vi "Main_v1.2.1.vi"() -> ()   [LabVIEW 2018]
uses:
  <vilib>/Utility/error.llb/DialogType.ctl
panel:
  out "字符串":string
  out "Progress Bar":i32(slide) max=135 scale=1.0..2026.0
  out "结果":T1(plugin-control)
  out "识别螺旋桨":T1(plugin-control)
  out "识别空泡":T1(plugin-control)
  in  "停止按钮":bool
  in  "等待时间（毫秒）":u32=100
  in  "打开按钮":bool
  # "空泡智能识别系统"
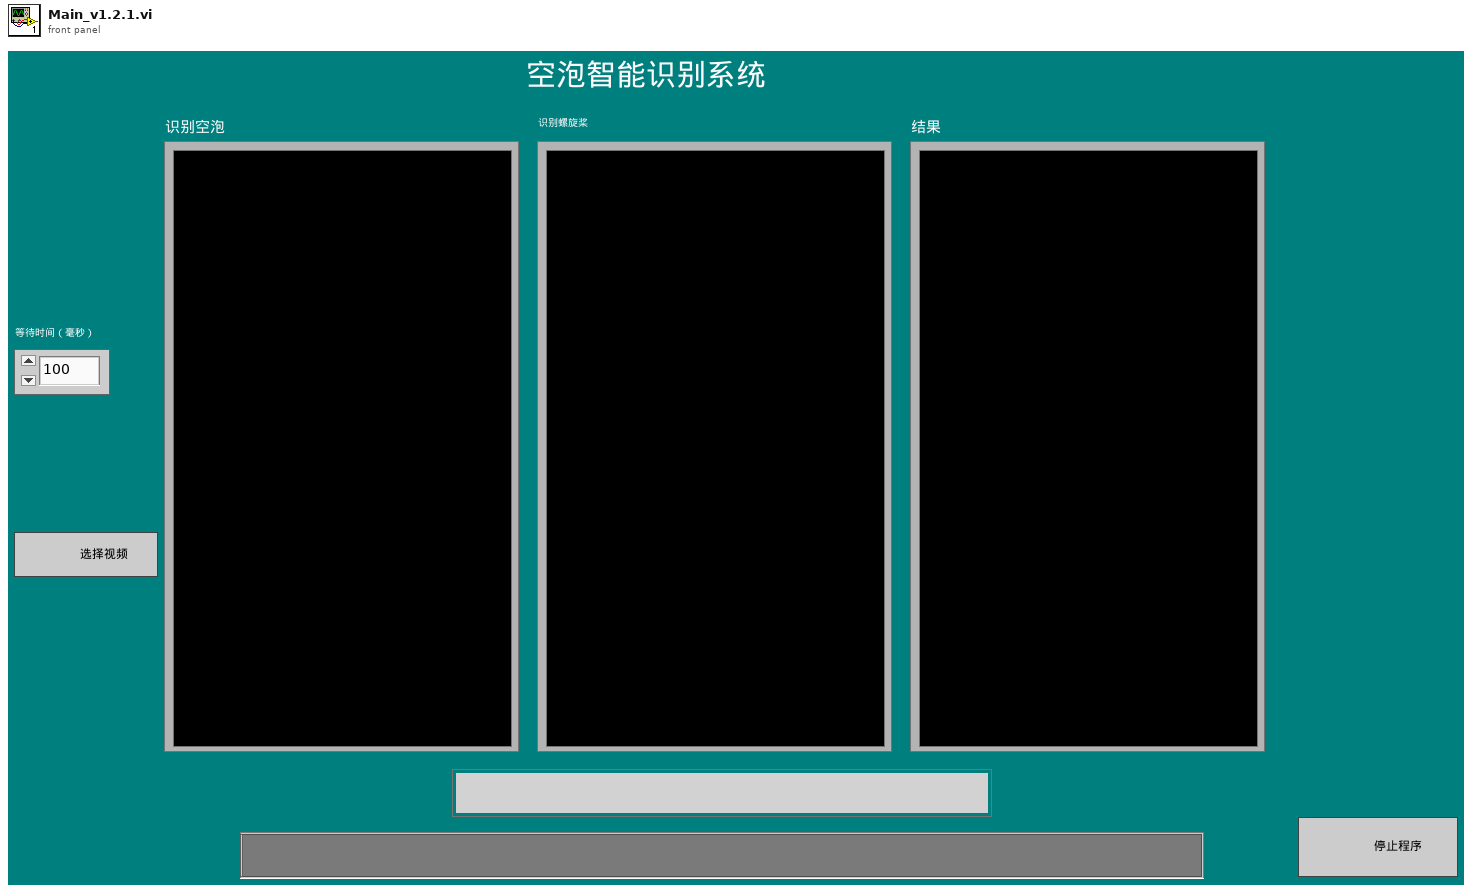
[diagram p1: front panel]
types:
  T1 = typedef "IMAQ Image.ctl" = refnum<image>
  T2 = cluster{"Desired Font (Application)":enum16{"User-specified Font", "Application Font", "System Font", "Dialog Font"}, "[User-specified Font]":cluster{"Font Name":string, "Size":i16, "Strikeout?":bool, "Italic?":bool, "Underline?":bool, "Outline?":bool, "Shadow?":bool, "Bold?":bool, "Rotation Angle":dbl}, "Horizontal Alignment":i16, "Vertical Alignment":i16}
  T3 = typedef "IMAQ AVI2 Refnum.ctl" = refnum<k20>
  T4 = typedef "Image Type" = u32
  T5 = cluster{"Width":u32, "Height":u32, "Frames Per Second":u32, "Codec":string, "Has Data":bool}
  T6 = typedef "DialogType.ctl" = u16
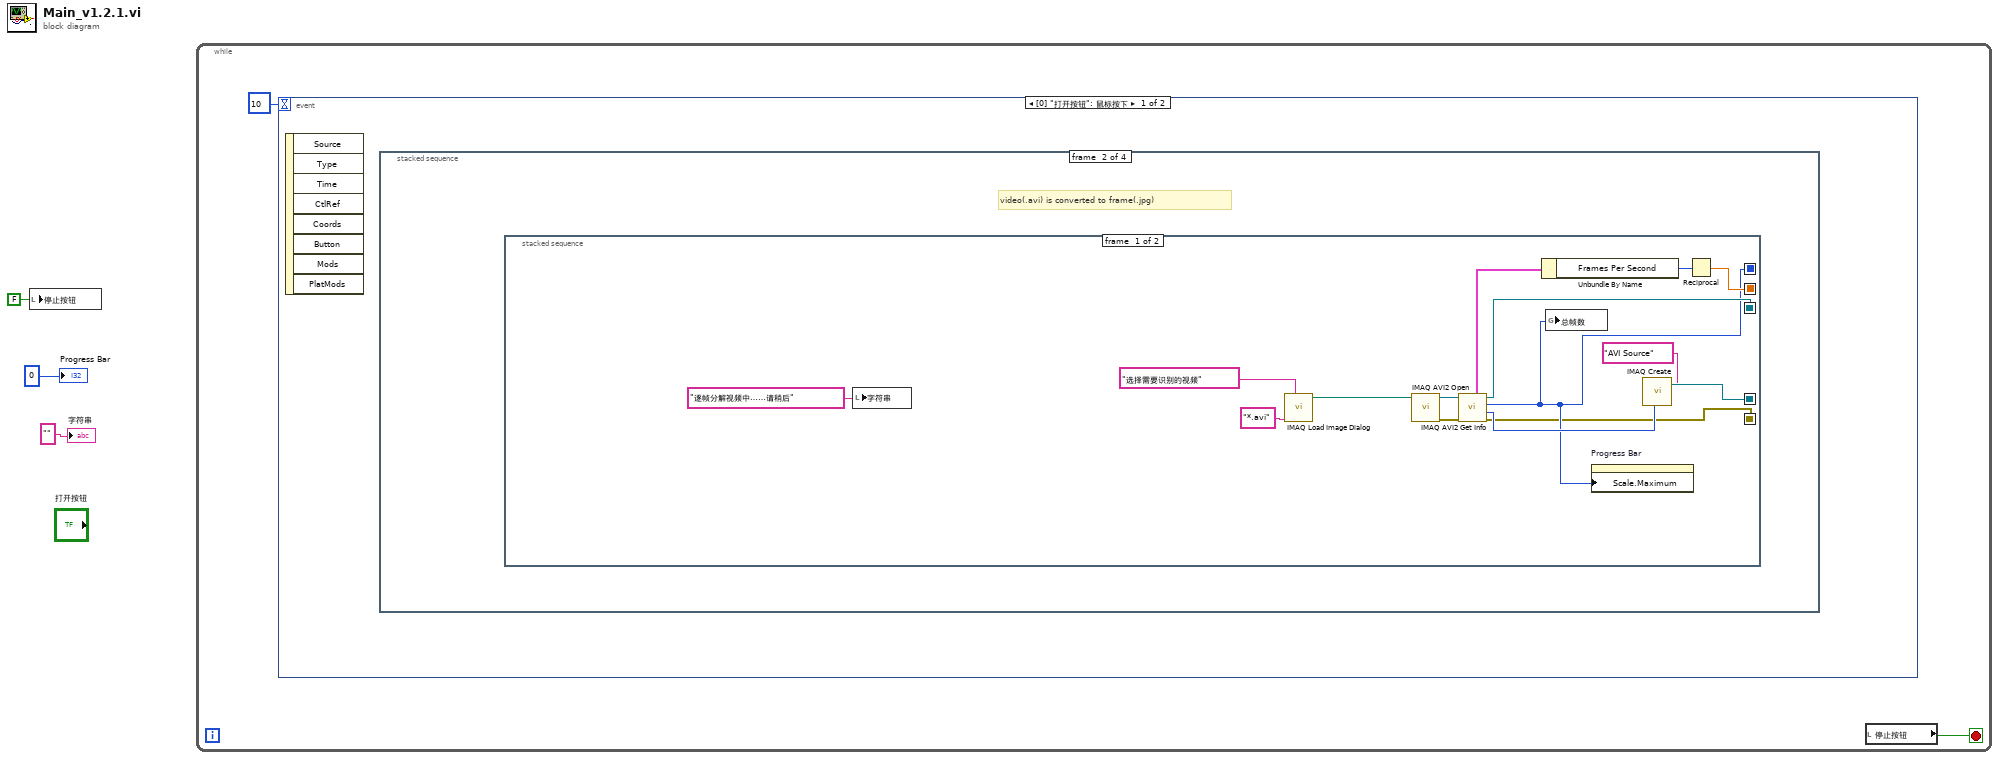
[diagram p0: block diagram]
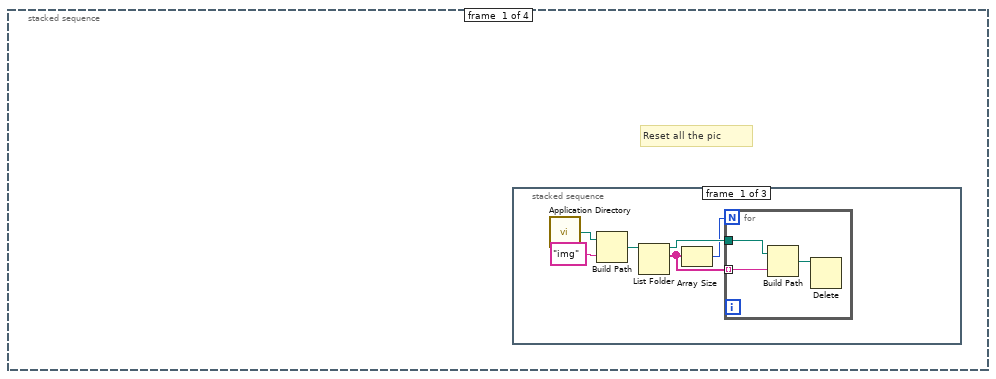
[diagram p2: hidden frame]
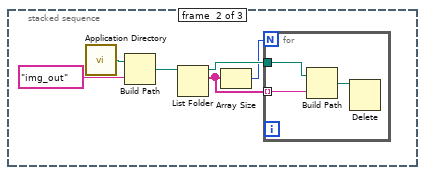
[diagram p3: hidden frame]
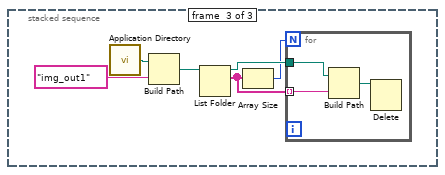
[diagram p4: hidden frame]
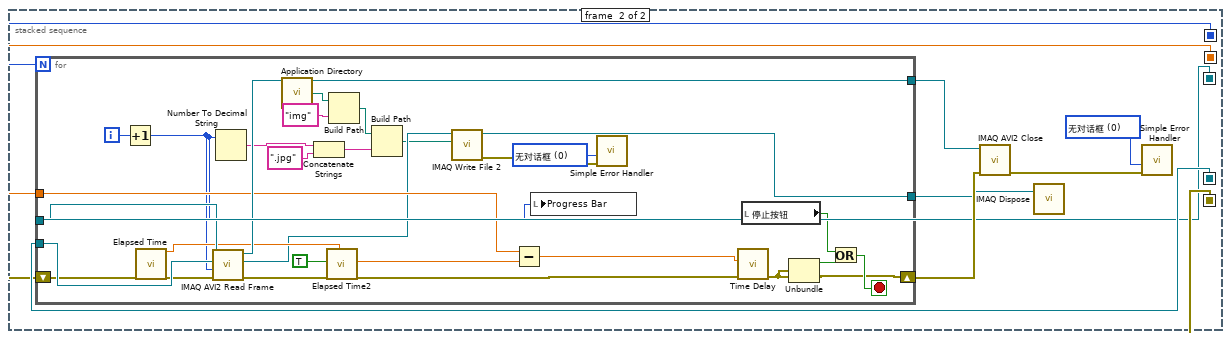
[diagram p5: hidden frame]
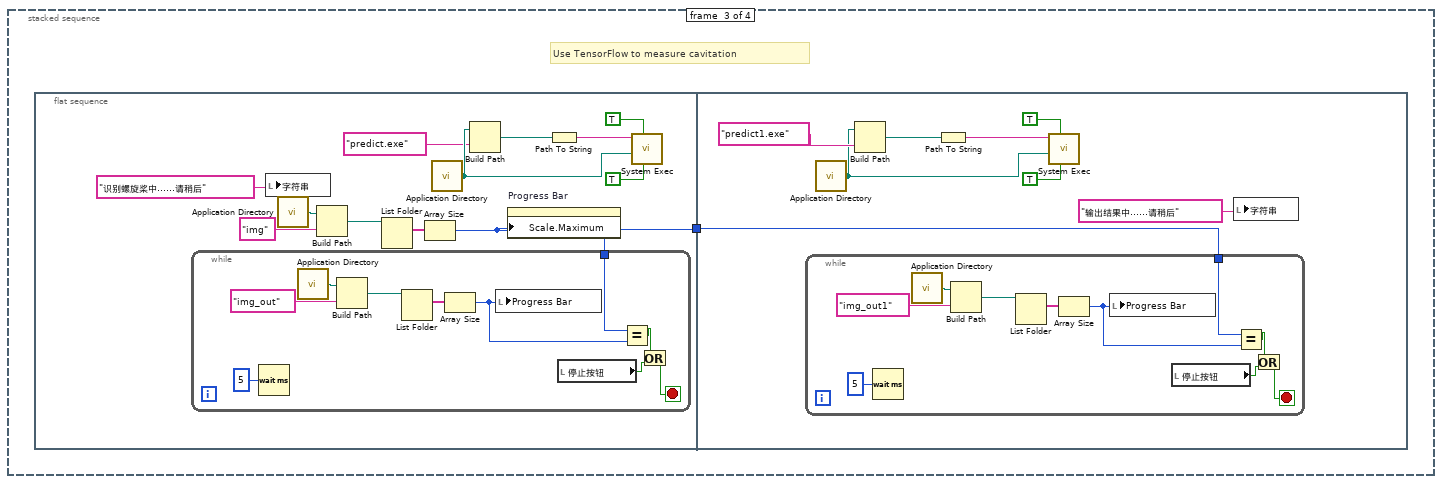
[diagram p6: hidden frame]
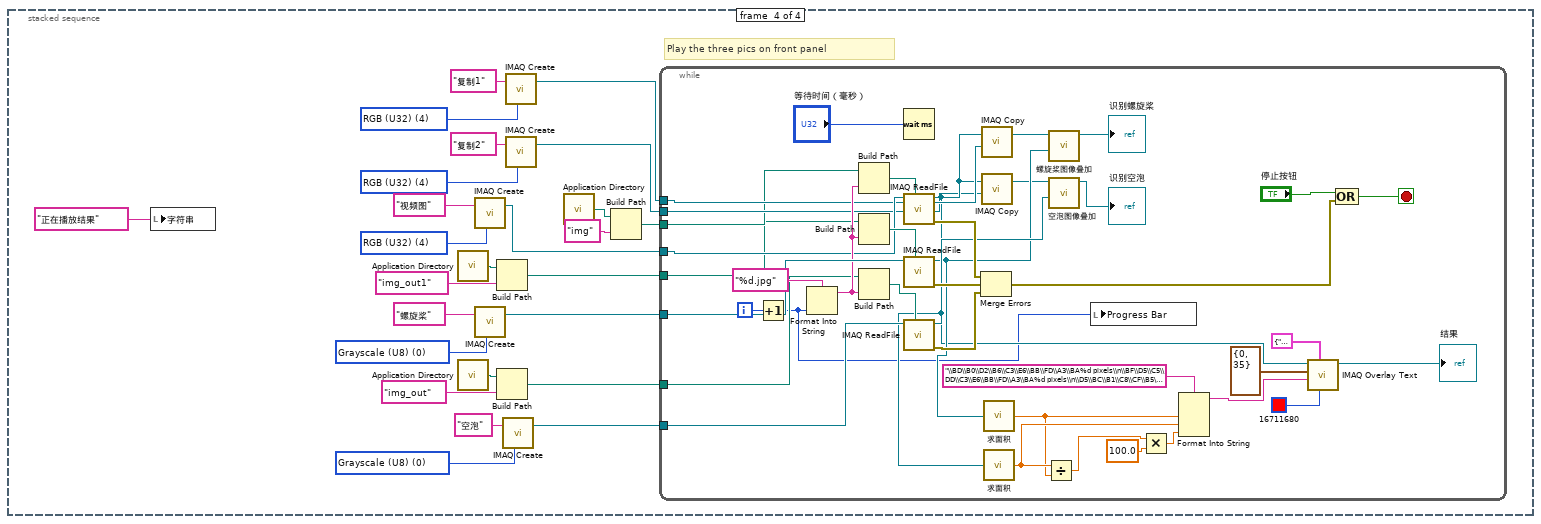
[diagram p7: hidden frame]
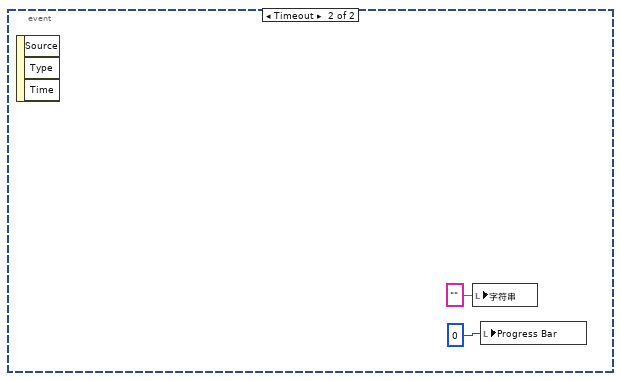
[diagram p8: hidden frame]
diagram:
  n1 = local write "停止按钮"(FALSE ("停止按钮")) -> ()
  n2 = while {
    stop <- w5 stop-if-true
    n3 = event shown="[0] \"打开按钮\": 鼠标按下" {
      selector: _ -> [_ _]
      dyn-events: _ -> [_ _]
      timeout: 10 -> [_ _]
      event "打开按钮": Mouse Down {
        n4 = event-data() -> ()  [unwired: 1 in, 8 out]
        n5 = stacked-sequence {
          frame #0 {
            # "Reset all the pic"
            n6 = stacked-sequence {
              frame #0 {
                n7 = call <vilib>:"Application Directory.vi"() -> ("Application Directory"=w10:path)
                n8 = Build Path(base path=w10, name or relative path="img" ("名称或相对路径")) -> (appended path=w8:path)
                n9 = List Folder(path=w8) -> (path out=w11:path, filenames=w6:string[])  [unwired: 3 in, 2 out]
                n10 = Array Size(array=w6) -> (size(s)=w7:i32)
                n11 = for {
                  N: w7 -> [_]
                  tunnel: w11 -> [w13]
                  tunnel: w6 -> [w12] mode=indexing
                  n12 = Build Path(base path=w13, name or relative path=w12) -> (appended path=w14:path)
                  n13 = Delete(path (use dialog)=w14) -> ()  [unwired: 4 in, 3 out]
                }
              }
              frame #1 {
                n14 = call <vilib>:"Application Directory.vi"() -> ("Application Directory"=w19:path)
                n15 = Build Path(base path=w19, name or relative path="img_out" ("名称或相对路径")) -> (appended path=w17:path)
                n16 = List Folder(path=w17) -> (path out=w20:path, filenames=w15:string[])  [unwired: 3 in, 2 out]
                n17 = Array Size(array=w15) -> (size(s)=w16:i32)
                n18 = for {
                  N: w16 -> [_]
                  tunnel: w20 -> [w22]
                  tunnel: w15 -> [w21] mode=indexing
                  n19 = Build Path(base path=w22, name or relative path=w21) -> (appended path=w23:path)
                  n20 = Delete(path (use dialog)=w23) -> ()  [unwired: 4 in, 3 out]
                }
              }
              frame #2 {
                n21 = call <vilib>:"Application Directory.vi"() -> ("Application Directory"=w28:path)
                n22 = Build Path(base path=w28, name or relative path="img_out1" ("名称或相对路径")) -> (appended path=w26:path)
                n23 = List Folder(path=w26) -> (path out=w29:path, filenames=w25:string[])  [unwired: 3 in, 2 out]
                n24 = Array Size(array=w25) -> (size(s)=w24:i32)
                n25 = for {
                  N: w24 -> [_]
                  tunnel: w29 -> [w31]
                  tunnel: w25 -> [w30] mode=indexing
                  n26 = Build Path(base path=w31, name or relative path=w30) -> (appended path=w32:path)
                  n27 = Delete(path (use dialog)=w32) -> ()  [unwired: 4 in, 3 out]
                }
              }
            }
          }
          frame #1 {
            # "video(.avi) is converted to frame(.jpg)"
            n28 = stacked-sequence {
              seq-local: [w35 _] -> [_ w49]
              seq-local: [w34 _] -> [_ w52]
              seq-local: [w44 _] -> [_ w53]
              seq-local: [w43 _] -> [_ w51]
              seq-local: [w40 _] -> [_ w50]
              frame #0 {
                n29 = local write "字符串"("逐帧分解视频中……请稍后" ("字符串")) -> ()
                n30 = call "IMAQ Load Image Dialog"("Prompt"="选择需要识别的视频" ("prompt"), "Pattern"="*.avi") -> ("Path"=w39:path)  [unwired: 7 in, 2 out]
                n31 = call "IMAQ AVI2 Open"("AVI File Path"=w39) -> ("error out"=w46:errorcluster, "AVI Refnum"=w45:T3)  [unwired: 2 in, 7 out]
                n32 = call "IMAQ AVI2 Get Info"("error in (no error)"=w46, "AVI Refnum"=w45) -> ("error out"=w34:errorcluster, "Image Type"=w42:T4, "Number of Frames"=w35:u32, "AVI Refnum (duplicate)"=w43:T3, "Frame Data"=w47:T5)  [unwired: 5 out]
                n33 = Unbundle By Name(w47) -> ("Frames Per Second"=w41:u32)
                n34 = global write "全局变量.vi" "总帧数"(w35) -> ()
                n35 = property on="Progress Bar" class="Slide (严格)"("Scale.Maximum"=w35) -> ()  [unwired: 2 in, 2 out]
                n36 = call "IMAQ Create"("Image Name"="AVI Source", "Image Type"=w42) -> ("New Image"=w44:T1)  [unwired: 2 in, 2 out]
                n37 = Reciprocal(x=w41) -> (1/x=w40:dbl)
              }
              frame #1 {
                w54 = T6 0 items=["无对话框", "确定信息", "继续或停止信息", "确定信息＋警告", "继续/停止+警告"] ("type of dialog (OK msg:1)")
                n38 = for "For循环" {
                  N: w49 -> [_]
                  tunnel: [w84] -> w57
                  tunnel: w51 -> [w86]
                  tunnel: w50 -> [w81]
                  shift-right: [w62] -> w56
                  shift-left: w52 -> [w83]
                  tunnel: w53 -> [w85]
                  tunnel: [w60] -> w48
                  i -> [w66]
                  stop <- w64 stop-if-true
                  w58 = T6 0 items=["无对话框", "确定信息", "继续或停止信息", "确定信息＋警告", "继续/停止+警告"] ("type of dialog (OK msg:1)")
                  n39 = Increment(x=w66) -> (x+1=w65:i32)
                  n40 = call "Elapsed Time"("error in (no error)"=w83) -> ("Present (s)"=w79:dbl, "error out"=w82:errorcluster)  [unwired: 11 in, 6 out]
                  n41 = call "IMAQ AVI2 Read Frame"("error in (no error)"=w82, "Frame Number"=w65, "Image"=w85, "AVI Refnum"=w86) -> ("error out"=w77:errorcluster, "Image Out"=w74:T1, "AVI Refnum (duplicate)"=w84:T3)  [unwired: 5 out]
                  n42 = Number To Decimal String(number=w65) -> (decimal integer string=w69:string)  [unwired: 1 in]
                  n43 = call <vilib>:"Application Directory.vi"() -> ("Application Directory"=w73:path)
                  n44 = Concatenate Strings(w69, ".jpg" ("字符串")) -> (w67:string)
                  n45 = call "Elapsed Time2"("Reset"=TRUE, "error in (no error)"=w77, "Set Start Time (s)"=w79) -> ("Elapsed Time (s)"=w76:dbl, "error out"=w75:errorcluster)  [unwired: 9 in, 6 out]
                  n46 = Build Path(base path=w73, name or relative path="img" ("名称或相对路径")) -> (appended path=w71:path)
                  n47 = Build Path(base path=w71, name or relative path=w67) -> (appended path=w70:path)
                  n48 = call-poly "IMAQ Write File 2"("File Path"=w70, "Image"=w74) -> ("error out"=w59:errorcluster, "Image Out (duplicate)"=w60:T1)  [unwired: 8 in]
                  n49 = Subtract(x=w81, y=w76) -> (x-y=w80:dbl)
                  n50 = local write "Progress Bar"(w65) -> ()
                  n51 = call <vilib>:"Simple Error Handler.vi"("type of dialog (OK msg:1)"=w58, "error in (no error)"=w59) -> ()  [unwired: 3 in, 5 out]
                  n52 = call "Time Delay"("error in (no error)"=w75, "Delay Time (s)"=w80) -> ("error out"=w62:errorcluster)  [unwired: 9 in]
                  n53 = local read "停止按钮"() -> (w63:bool)
                  n54 = Unbundle(w62) -> ("status"=w61:bool)  [unwired: 2 out]
                  n55 = Or(x=w63, y=w61) -> (x .or. y?=w64:bool)
                }
                n56 = call "IMAQ AVI2 Close"("error in (no error)"=w56, "AVI Refnum"=w57) -> ("error out"=w55:errorcluster)  [unwired: 9 out]
                n57 = call "IMAQ Dispose"("Image"=w48) -> ()  [unwired: 2 in, 4 out]
                n58 = call <vilib>:"Simple Error Handler.vi"("type of dialog (OK msg:1)"=w54, "error in (no error)"=w55) -> ()  [unwired: 8 out]
              }
            }
          }
          frame #2 {
            # "Use TensorFlow to measure cavitation"
            n59 = flat-sequence {
              tunnel: [w88] -> w87
              tunnel: w87 -> [w110]
              frame #0 {
                n60 = local write "字符串"("识别螺旋桨中……请稍后" ("字符串")) -> ()
                n61 = call <vilib>:"Application Directory.vi"() -> ("Application Directory"=w90:path)
                n62 = Build Path(base path=w90, name or relative path="img" ("名称或相对路径")) -> (appended path=w91:path)
                n63 = List Folder(path=w91) -> (filenames=w89:string[])  [unwired: 3 in, 3 out]
                n64 = Array Size(array=w89) -> (size(s)=w88:i32)
                n65 = while {
                  tunnel: w88 -> [w103]
                  stop <- w100 stop-if-true
                  n66 = Wait (ms)(milliseconds to wait=u32 5 ("等待时间（毫秒）")) -> ()  [unwired: 1 out]
                  n67 = call <vilib>:"Application Directory.vi"() -> ("Application Directory"=w108:path)
                  n68 = Build Path(base path=w108, name or relative path="img_out" ("名称或相对路径")) -> (appended path=w107:path)
                  n69 = List Folder(path=w107) -> (filenames=w109:string[])  [unwired: 3 in, 3 out]
                  n70 = Array Size(array=w109) -> (size(s)=w104:i32)
                  n71 = local write "Progress Bar"(w104) -> ()
                  n72 = local read "停止按钮"() -> (w102:bool)
                  n73 = Equal?(x=w103, y=w104) -> (x = y?=w101:bool)
                  n74 = Or(x=w101, y=w102) -> (x .or. y?=w100:bool)
                }
                n75 = call <vilib>:"Application Directory.vi"() -> ("Application Directory"=w97:path)
                n76 = Build Path(base path=w97, name or relative path="predict.exe" ("名称或相对路径")) -> (appended path=w95:path)
                n77 = property on="Progress Bar" class="Slide (严格)"("Scale.Maximum"=w88) -> ()  [unwired: 2 in, 2 out]
                n78 = Path To String(path=w95) -> (string=w94:string)
                n79 = call <vilib>:"System Exec.vi"("run minimized? (F)"=TRUE, "wait until completion? (T)"=TRUE, "working directory"=w97, "command line"=w94) -> ()  [unwired: 4 in, 4 out]
              }
              frame #1 {
                n80 = while {
                  tunnel: w110 -> [w121]
                  stop <- w118 stop-if-true
                  n81 = Wait (ms)(milliseconds to wait=u32 5 ("等待时间（毫秒）")) -> ()  [unwired: 1 out]
                  n82 = call <vilib>:"Application Directory.vi"() -> ("Application Directory"=w126:path)
                  n83 = Build Path(base path=w126, name or relative path="img_out1" ("名称或相对路径")) -> (appended path=w125:path)
                  n84 = List Folder(path=w125) -> (filenames=w127:string[])  [unwired: 3 in, 3 out]
                  n85 = Array Size(array=w127) -> (size(s)=w122:i32)
                  n86 = local write "Progress Bar"(w122) -> ()
                  n87 = local read "停止按钮"() -> (w120:bool)
                  n88 = Equal?(x=w121, y=w122) -> (x = y?=w119:bool)
                  n89 = Or(x=w119, y=w120) -> (x .or. y?=w118:bool)
                }
                n90 = call <vilib>:"Application Directory.vi"() -> ("Application Directory"=w112:path)
                n91 = Build Path(base path=w112, name or relative path="predict1.exe" ("名称或相对路径")) -> (appended path=w114:path)
                n92 = Path To String(path=w114) -> (string=w113:string)
                n93 = call <vilib>:"System Exec.vi"("run minimized? (F)"=TRUE, "wait until completion? (T)"=TRUE, "working directory"=w112, "command line"=w113) -> ()  [unwired: 4 in, 4 out]
                n94 = local write "字符串"("输出结果中……请稍后" ("字符串")) -> ()
              }
            }
          }
          frame #3 {
            w140 = T4 4 items=["Grayscale (U8)", "Grayscale (I16)", "Grayscale (SGL)", "Complex (CSG)", "RGB (U32)", "HSL (U32)", "RGB (U64)", "Grayscale (U16)"] ("Image Type")
            w143 = T4 4 items=["Grayscale (U8)", "Grayscale (I16)", "Grayscale (SGL)", "Complex (CSG)", "RGB (U32)", "HSL (U32)", "RGB (U64)", "Grayscale (U16)"] ("Image Type")
            w146 = T4 0 items=["Grayscale (U8)", "Grayscale (I16)", "Grayscale (SGL)", "Complex (CSG)", "RGB (U32)", "HSL (U32)", "RGB (U64)", "Grayscale (U16)"] ("Image Type")
            w149 = T4 0 items=["Grayscale (U8)", "Grayscale (I16)", "Grayscale (SGL)", "Complex (CSG)", "RGB (U32)", "HSL (U32)", "RGB (U64)", "Grayscale (U16)"] ("Image Type")
            w151 = T4 4 items=["Grayscale (U8)", "Grayscale (I16)", "Grayscale (SGL)", "Complex (CSG)", "RGB (U32)", "HSL (U32)", "RGB (U64)", "Grayscale (U16)"] ("Image Type")
            # "Play the three pics on front panel"
            n95 = local write "字符串"("正在播放结果" ("字符串")) -> ()
            n96 = call <vilib>:"Application Directory.vi"() -> ("Application Directory"=w131:path)
            n97 = call <vilib>:"Application Directory.vi"() -> ("Application Directory"=w133:path)
            n98 = call "IMAQ Create"("Image Name"="视频图", "Image Type"=w151) -> ("New Image"=w150:T1)  [unwired: 3 in, 1 out]
            n99 = call "IMAQ Create"("Image Name"="螺旋桨", "Image Type"=w149) -> ("New Image"=w144:T1)  [unwired: 3 in, 1 out]
            n100 = Build Path(base path=w131, name or relative path="img_out1" ("名称或相对路径")) -> (appended path=w129:path)
            n101 = Build Path(base path=w133, name or relative path="img_out" ("名称或相对路径")) -> (appended path=w132:path)
            n102 = call "IMAQ Create"("Image Name"="空泡", "Image Type"=w146) -> ("New Image"=w145:T1)  [unwired: 3 in, 1 out]
            n103 = call "IMAQ Create"("Image Name"="复制1", "Image Type"=w143) -> ("New Image"=w139:T1)  [unwired: 3 in, 1 out]
            n104 = call "IMAQ Create"("Image Name"="复制2", "Image Type"=w140) -> ("New Image"=w138:T1)  [unwired: 3 in, 1 out]
            n105 = call <vilib>:"Application Directory.vi"() -> ("Application Directory"=w137:path)
            n106 = Build Path(base path=w137, name or relative path="img" ("名称或相对路径")) -> (appended path=w135:path)
            n107 = while {
              tunnel: w150 -> [w164]
              tunnel: w145 -> [w186]
              tunnel: w144 -> [w185]
              tunnel: w139 -> [w162]
              tunnel: w138 -> [w160]
              tunnel: w135 -> [w156]
              tunnel: w132 -> [w155]
              tunnel: w129 -> [w154]
              i -> [w175]
              stop <- w168 stop-if-true
              n108 = Increment(x=w175) -> (x+1=w153:i32)
              n109 = Format Into String(format string="%d.jpg" ("格式字符串"), w153) -> (resulting string=w174:string)  [unwired: 2 in, 1 out]
              n110 = Build Path(base path=w156, name or relative path=w174) -> (appended path=w187:path)
              n111 = Build Path(base path=w154, name or relative path=w174) -> (appended path=w184:path)
              n112 = Build Path(base path=w155, name or relative path=w174) -> (appended path=w183:path)
              n113 = Wait (ms)(milliseconds to wait="等待时间（毫秒）") -> ()  [unwired: 1 out]
              n114 = call "IMAQ ReadFile"("File Path"=w187, "Image"=w164) -> ("error out"=w171:errorcluster, "Image Out"=w161:T1)  [unwired: 5 in, 3 out]
              n115 = call "IMAQ ReadFile"("File Path"=w184, "Image"=w185) -> ("error out"=w170:errorcluster, "Image Out"=w163:T1)  [unwired: 5 in, 3 out]
              n116 = call "IMAQ ReadFile"("File Path"=w183, "Image"=w186) -> ("error out"=w169:errorcluster, "Image Out"=w166:T1)  [unwired: 5 in, 3 out]
              n117 = Merge Errors(w171, w170, w169) -> (w172:errorcluster)
              n118 = call "IMAQ Copy"("Image Dst"=w162, "Image Src"=w161) -> ("Image Dst Out"=w158:T1)  [unwired: 4 in, 1 out]
              n119 = call "IMAQ Copy"("Image Dst"=w160, "Image Src"=w161) -> ("Image Dst Out"=w159:T1)  [unwired: 4 in, 1 out]
              n120 = call "求面积.vi"("Image"=w163) -> ("数值输入控件"=w181:dbl)
              n121 = call "求面积.vi"("Image"=w166) -> ("数值输入控件"=w182:dbl)
              n122 = Divide(x=w182, y=w181) -> (x/y=w180:dbl)
              n123 = call "螺旋桨图像叠加.vi"("Image Src A"=w163, "Image Src"=w158) -> ("Image Dst Out"=→"识别螺旋桨":T1)  [unwired: 9 in]
              n124 = call "空泡图像叠加.vi"("Image Src A"=w166, "Image Src"=w159) -> ("Image Dst Out"=→"识别空泡":T1)  [unwired: 9 in]
              n125 = local write "Progress Bar"(w153) -> ()
              n126 = Multiply(x=w180, y=100.0) -> (x*y=w178:dbl)
              n127 = Format Into String(format string="\\BD\\B0\\D2\\B6\\C3\\E6\\BB\\FD\\A3\\BA%d pixels\\n\\BF\\D5\\C5\\DD\\C3\\E6\\BB\\FD\\A3\\BA%d pixels\\n\\D5\\BC\\B1\\C8\\CF\\B5\\CA\\FD\\A3\\BA%1.2f %%" ("初始字符串"), w181, w182, w178) -> (resulting string=w189:string)  [unwired: 2 in, 1 out]
              n128 = call "IMAQ Overlay Text"("Text Color (black)"=u32 16711680, "Font, Size & Style"=T2 {"Desired Font (Application)"=enum."User-specified Font", "[User-specified Font]"={"Font Name"="", "Size"=30, "Strikeout?"=FALSE, "Italic?"=FALSE, "Underline?"=FALSE, "Outline?"=FALSE, "Shadow?"=FALSE, "Bold?"=FALSE, "Rotation Angle"=0.0}, "Horizontal Alignment"=0, "Vertical Alignment"=0}, "String"=w189, "Origin"=cluster{"X":i32, "Y":i32} {"X"=0, "Y"=35}, "Image"=w161) -> ("Image Out"=→"结果":T1)  [unwired: 5 in, 1 out]
              n129 = Compound Arithmetic op=OR("停止按钮", w172) -> (w168:bool)
            }
          }
        }
      }
      event Timeout {
        n130 = event-data() -> ()  [unwired: 1 in, 3 out]
        n131 = local write "字符串"("" ("字符串")) -> ()
        n132 = local write "Progress Bar"(0 ("Progress Bar")) -> ()
      }
    }
    n133 = local read "停止按钮"() -> (w5:bool)
  }
  "Progress Bar" <- 0 ("Progress Bar")
  "字符串" <- "" ("字符串")
